vi "initCAN.vi"(1 "Baud Rate":T2(ring), 2 "CPOL":bool, 3 "MXP Port":enum16{"A", "B"}(ring)) -> (0 "SPI Config Out":T1)   [LabVIEW 2019]
uses:
  SPI/SPI Config.ctl
panel:
  in  "SPI Config In":T1
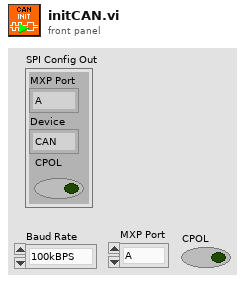
[diagram p1: front panel]
types:
  T1 = typedef "SPI Config.ctl" = cluster{"MXP Port":enum16{"A", "B"}, "Device":enum16{"CAN", "ENC", "IMU1", "IMU2"}, "CPOL":bool}
  T2 = enum16{"100kBPS", "250kBPS", "500kBPS", "1000kBPS"}
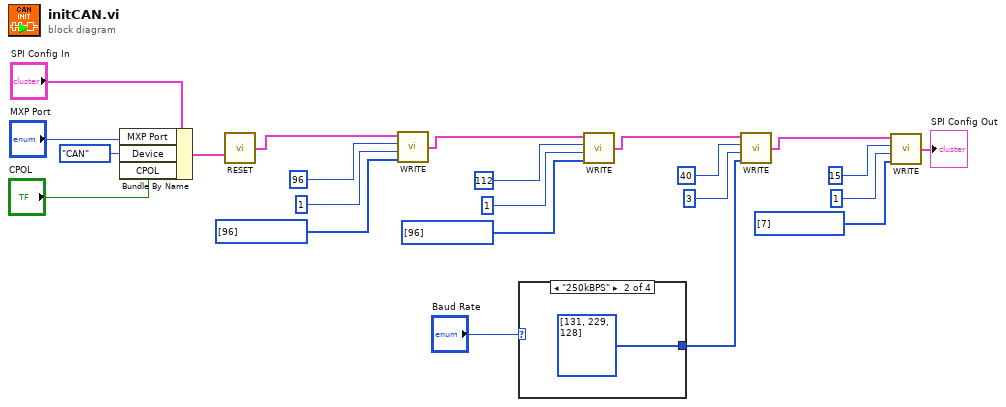
[diagram p0: block diagram]
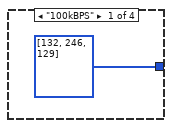
[diagram p2: hidden frame]
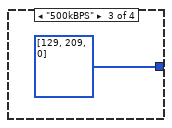
[diagram p3: hidden frame]
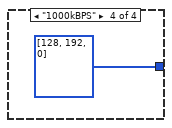
[diagram p4: hidden frame]
diagram:
  n1 = Bundle By Name(cluster="SPI Config In", "MXP Port"="MXP Port", "Device"=enum16{"CAN", "ENC", "IMU1", "IMU2"}."CAN", "CPOL"="CPOL") -> (w2:T1)
  n2 = call "RESET.vi"("SPI Config In"=w2) -> ("SPI Config Out"=w16:T1)
  n3 = call "WRITE.vi"("Data to Write"=u8[] [96], "Frames to Write"=u8 1, "Starting Address"=u8 96, "SPI Config In"=w16) -> ("SPI Config Out"=w17:T1)
  n4 = case shown="\"250kBPS\"" "Baud Rate" {
    tunnel: [i16[] [132, 246, 129] i16[] [131, 229, 128] i16[] [129, 209, 0] i16[] [128, 192, 0]] -> w6
    frame "100kBPS" {
    }
    frame "250kBPS" {
    }
    frame "500kBPS" {
    }
    frame "1000kBPS" {
    }
  }
  n5 = call "WRITE.vi"("Data to Write"=u8[] [96], "Frames to Write"=u8 1, "Starting Address"=u8 112, "SPI Config In"=w17) -> ("SPI Config Out"=w13:T1)
  n6 = call "WRITE.vi"("Data to Write"=w6, "Frames to Write"=u8 3, "Starting Address"=u8 40, "SPI Config In"=w13) -> ("SPI Config Out"=w12:T1)
  n7 = call "WRITE.vi"("Data to Write"=u8[] [7], "Frames to Write"=u8 1, "Starting Address"=u8 15, "SPI Config In"=w12) -> ("SPI Config Out"=→"SPI Config Out":T1)
